vi "Example Command to gRPC.vi"(8 "error in (no error)":errorcluster, 11 "CIFPlugin in":refnum<class "Template_Plugin.lvclass">) -> (0 "error out":errorcluster, 3 "CIFPlugin out":refnum<class "Template_Plugin.lvclass">)   [LabVIEW 2021, in "Template_Plugin.lvclass"]
uses:
  Template_Plugin.lvclass
  Template_Plugin.lvclass/Template_Plugin.ctl
  Common/Typedef/OOB Comm/To gRPC Command Payload.ctl
  Common/Typedef/OOB Comm/To gRPC Command.ctl
  Common/Typedef/OOB Comm/To gRPC Command Data.ctl
  68de193c-236d-478b-a1f8-a234f3c413fe.vi
  <vilib>/CIF Foundation/CIF CIPC/SubVIs/Check Error.vi
  <vilib>/CIF Foundation/CIF CIPC/SubVIs/Notify Of New Write.vi
  <vilib>/CIF Foundation/CIF CIPC/SubVIs/Get dll Path.vi
  <vilib>/CIF Foundation/CIF CIPC/SubVIs/Get Element Write Position.vi
  <vilib>/CIF Foundation/CIF CIPC/SubVIs/Get Element Info Variant.vi
  <vilib>/Utility/error.llb/Trim Whitespace.vi
  <vilib>/Utility/error.llb/Error Cluster From Error Code.vi
  Common/Template_Common.lvlib
  43c951f1-2923-4d19-899c-527205ee8bff.vi
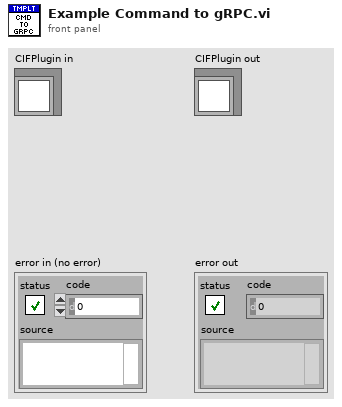
[diagram p1: front panel]
types:
  T1 = typedef "Template_Common.lvlib/To gRPC Command Payload.ctl" = cluster{"-> gRPC Command":T2, "-> gRPC Data":T3}
  T2 = typedef "Template_Common.lvlib/To gRPC Command.ctl" = enum16{"Read Data", "Read DVR Data"}
  T3 = typedef "Template_Common.lvlib/To gRPC Command Data.ctl" = cluster{"Cmd Data 1 -> gRPC":i32}
  T4 = typedef "Template_Common.lvlib/To gRPC DVR Data.ctl" = cluster{"Data 1 DVR -> gRPC ":i32}
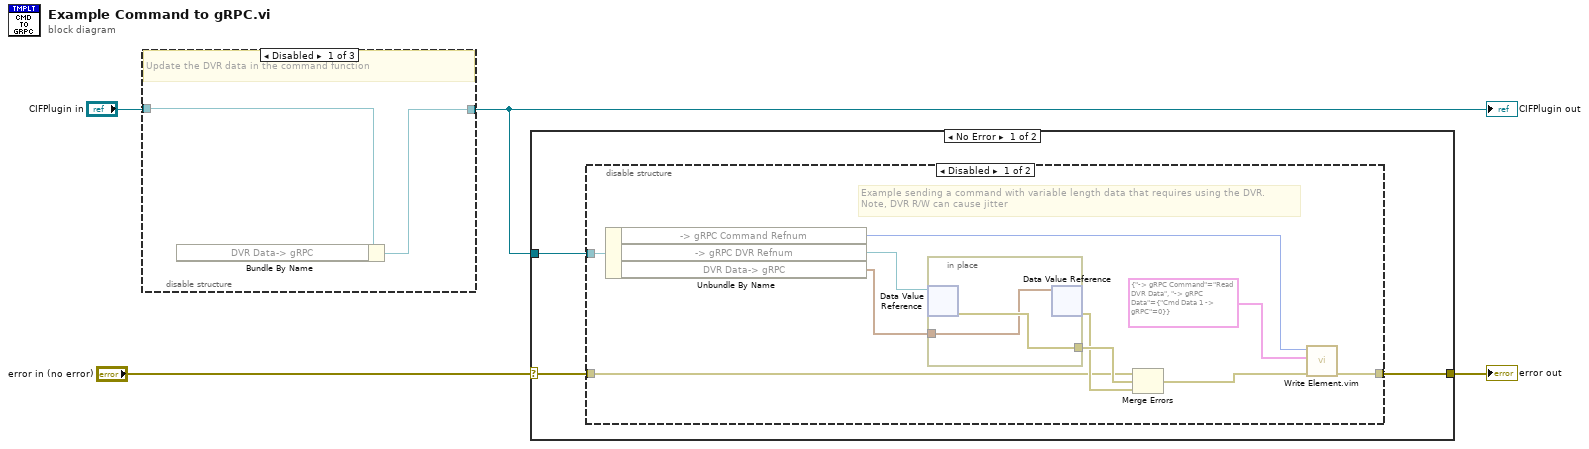
[diagram p0: block diagram]
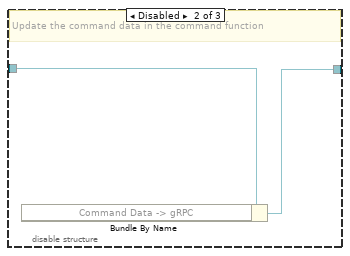
[diagram p2: hidden frame]
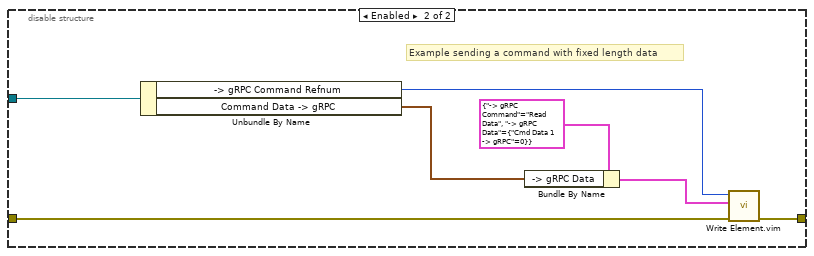
[diagram p4: hidden frame]
diagram:
  n1 = disable-structure shown="Disabled" {
    disable-tunnel: "CIFPlugin in" -> [w6 w8 w9]
    disable-tunnel: [w5 w7 w9] -> w1
    frame Disabled {
      # "Update the DVR data in the command function"
      n2 = Bundle By Name(cluster=w6) -> (w5:refnum<class "Template_Plugin.lvclass">)  [unwired: 1 in]
    }
    frame Disabled {
      # "Update the command data in the command function"
      n3 = Bundle By Name(cluster=w8) -> (w7:refnum<class "Template_Plugin.lvclass">)  [unwired: 1 in]
    }
    frame Enabled {
      # "The new data was previously written into the class."
    }
  }
  "CIFPlugin out" <- w1
  n4 = case shown="No Error" "error in (no error)" {
    selector: "error in (no error)" -> [w11 w32]
    tunnel: [w10 w32] -> w2
    tunnel: w1 -> [w12 _]
    frame No Error {
      n5 = disable-structure shown="Disabled" {
        disable-tunnel: w12 -> [w17 w30]
        disable-tunnel: w11 -> [w16 w28]
        disable-tunnel: [w15 w29] -> w10
        frame Disabled {
          # "Example sending a command with variable length data that requires using the DVR.\nNote, DVR R/W can cause jitter"
          n6 = Unbundle By Name(w17) -> ("-> gRPC Command Refnum"=w19:u64, "-> gRPC DVR Refnum"=w22:refnum<data-value>, "DVR Data-> gRPC"=w13:T4)
          n7 = in-place {
            in-place-border: [w24] -> w20
            in-place-border: w13 -> [w23]
            n8 = in-place-dvr #1(w22) -> (w24:errorcluster)  [unwired: 1 out]
            n9 = in-place-dvr #1(w23) -> (w18:errorcluster)  [unwired: 1 out]
          }
          n10 = Merge Errors(w16, w20, w18) -> (w21:errorcluster)
          n11 = call "Write Element.vim"("error in (no error)"=w21, "Data in"=T1 {"-> gRPC Command"=enum."Read DVR Data", "-> gRPC Data"={"Cmd Data 1 -> gRPC"=0}} ("-> gRPC Payload"), "CIPC Reference in"=w19) -> ("error out"=w15:errorcluster)  [unwired: 5 in, 3 out]
        }
        frame Enabled {
          # "Example sending a command with fixed length data"
          n12 = Unbundle By Name(w30) -> ("-> gRPC Command Refnum"=w31:u64, "Command Data -> gRPC"=w26:T3)
          n13 = Bundle By Name(cluster=T1 {"-> gRPC Command"=enum."Read Data", "-> gRPC Data"={"Cmd Data 1 -> gRPC"=0}} ("-> gRPC Payload"), "-> gRPC Data"=w26) -> (w27:T1)
          n14 = call "Write Element.vim"("error in (no error)"=w28, "Data in"=w27, "CIPC Reference in"=w31) -> ("error out"=w29:errorcluster)  [unwired: 5 in, 3 out]
        }
      }
    }
    frame Error {
    }
  }
  "error out" <- w2
